vi "Splay Bind.vi"(9 "Button Input":bool, 10 "Pull Solenoid Ref":string, 11 "Push Solenoid Ref":string) -> ()   [LabVIEW 2018]
uses:
  <vilib>/Rock Robotics/WPI/Solenoid/Deprecated/WPI_SolenoidGetBool.vi
  <vilib>/Rock Robotics/WPI/Solenoid/Deprecated/WPI_SolenoidSetBool.vi
  <vilib>/Rock Robotics/WPI/Solenoid/WPI_SolenoidSetEnum.vi
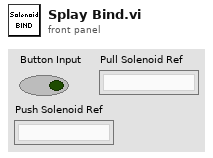
[diagram p1: front panel]
types:
  T1 = typedef "WPI_SolenoidDevRef.ctl" = cluster{"DevStatus":errorcluster, "Pneumatics Control Module":u8, "Forward Solenoid Channel":T2, "Reverse Solenoid Channel":T2}
  T2 = typedef "WPI_SolenoidChannel.ctl" = enum8{"Solenoid 0", "Solenoid 1", "Solenoid 2", "Solenoid 3", "Solenoid 4", "Solenoid 5", "Solenoid 6", "Solenoid 7", "Invalid"}
  T3 = typedef "WPI_SolenoidValue.ctl" = enum16{"Off", "On", "Forward", "Reverse"}
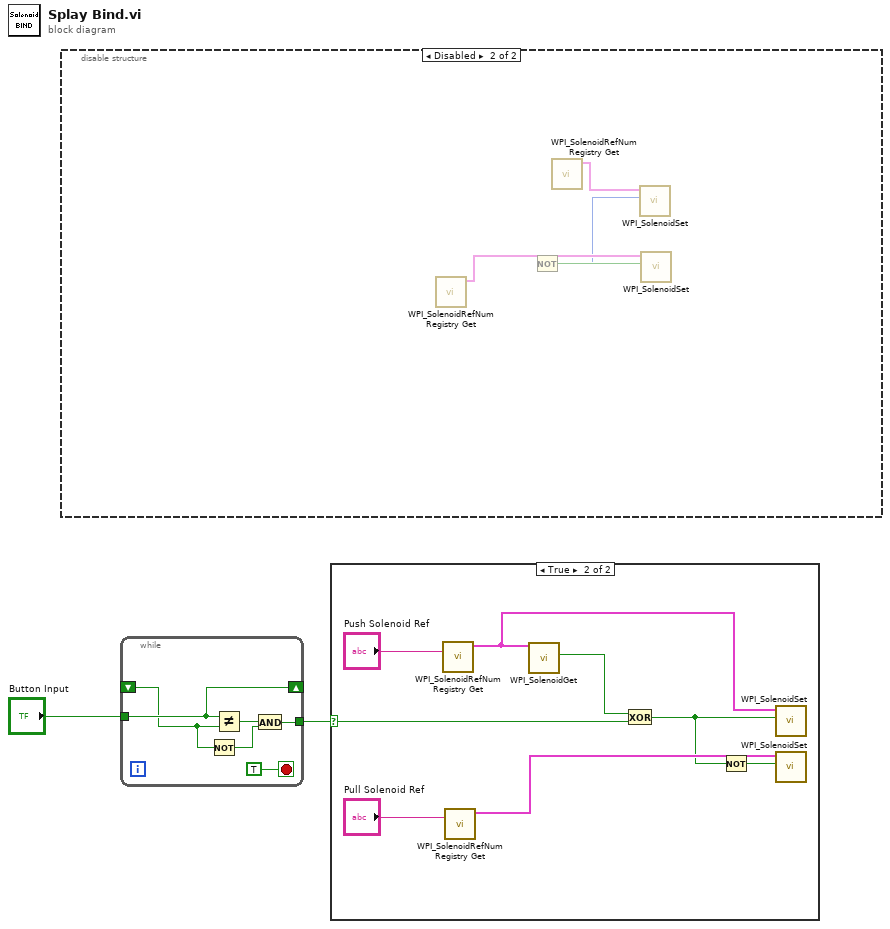
[diagram p0: block diagram]
diagram:
  n1 = disable-structure shown="Disabled" {
    frame Enabled {
    }
    frame Disabled {
      n2 = call <vilib>:"WPI_SolenoidRefNum Registry Get.vi"() -> ("SolenoidDevRef"=w7:T1, "refnum name"=w3:string)  [unwired: 9 in, 1 out]
      n3 = call <vilib>:"WPI_SolenoidRefNum Registry Get.vi"() -> ("SolenoidDevRef"=w6:T1, "refnum name"=w4:string)  [unwired: 9 in, 1 out]
      n4 = call-poly <vilib>:"WPI_SolenoidSet.vi"("SolenoidDevRef"=w6) -> ("Value"=w5:T3)  [unwired: 8 in, 2 out]
      n5 = Not(x=w5) -> (.not. x?=w8:bool)
      n6 = call-poly <vilib>:"WPI_SolenoidSet.vi"("Value"=w8, "SolenoidDevRef"=w7) -> ()  [unwired: 8 in, 2 out]
    }
  }
  n7 = while {
    shift-right: [w14] -> _
    shift-left: _ -> [w12]
    tunnel: "Button Input" -> [w14]
    tunnel: [w11] -> w2
    stop <- TRUE stop-if-true
    n8 = Not(x=w12) -> (.not. x?=w9:bool)
    n9 = Not Equal?(x=w14, y=w12) -> (x != y?=w10:bool)
    n10 = And(x=w10, y=w9) -> (x .and. y?=w11:bool)
  }
  n11 = case shown="True" w2 {
    selector: w2 -> [_ w19]
    frame False {
    }
    frame True {
      n12 = call <vilib>:"WPI_SolenoidRefNum Registry Get.vi"("refnum name"="Push Solenoid Ref") -> ("SolenoidDevRef"=w20:T1)  [unwired: 9 in, 1 out]
      n13 = call <vilib>:"WPI_SolenoidRefNum Registry Get.vi"("refnum name"="Pull Solenoid Ref") -> ("SolenoidDevRef"=w21:T1)  [unwired: 9 in, 1 out]
      n14 = call-poly <vilib>:"WPI_SolenoidGet.vi"("SolenoidDevRef"=w20) -> ("Value"=w22:bool)  [unwired: 8 in, 2 out]
      n15 = Exclusive Or(1:w19, 2:w22) -> (0:w15:bool)
      n16 = Not(x=w15) -> (.not. x?=w16:bool)
      n17 = call-poly <vilib>:"WPI_SolenoidSet.vi"("Value"=w15, "SolenoidDevRef"=w20) -> ()  [unwired: 8 in, 2 out]
      n18 = call-poly <vilib>:"WPI_SolenoidSet.vi"("Value"=w16, "SolenoidDevRef"=w21) -> ()  [unwired: 8 in, 2 out]
    }
  }
